vi "Drive Ramp.vi"(8 "Deadband":dbl, 9 "Ramp Value":dbl, 10 "Control Input":dbl, 11 "Previous Value":dbl) -> (3 "Next Value":dbl)   [LabVIEW 2012]
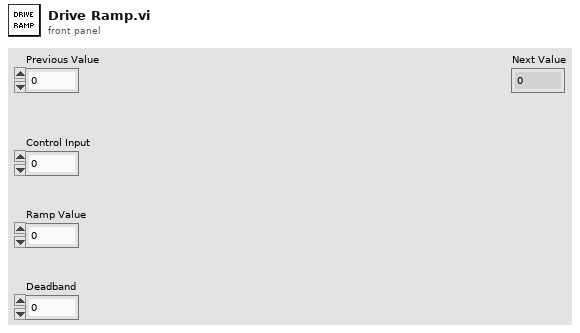
[diagram p1: front panel]
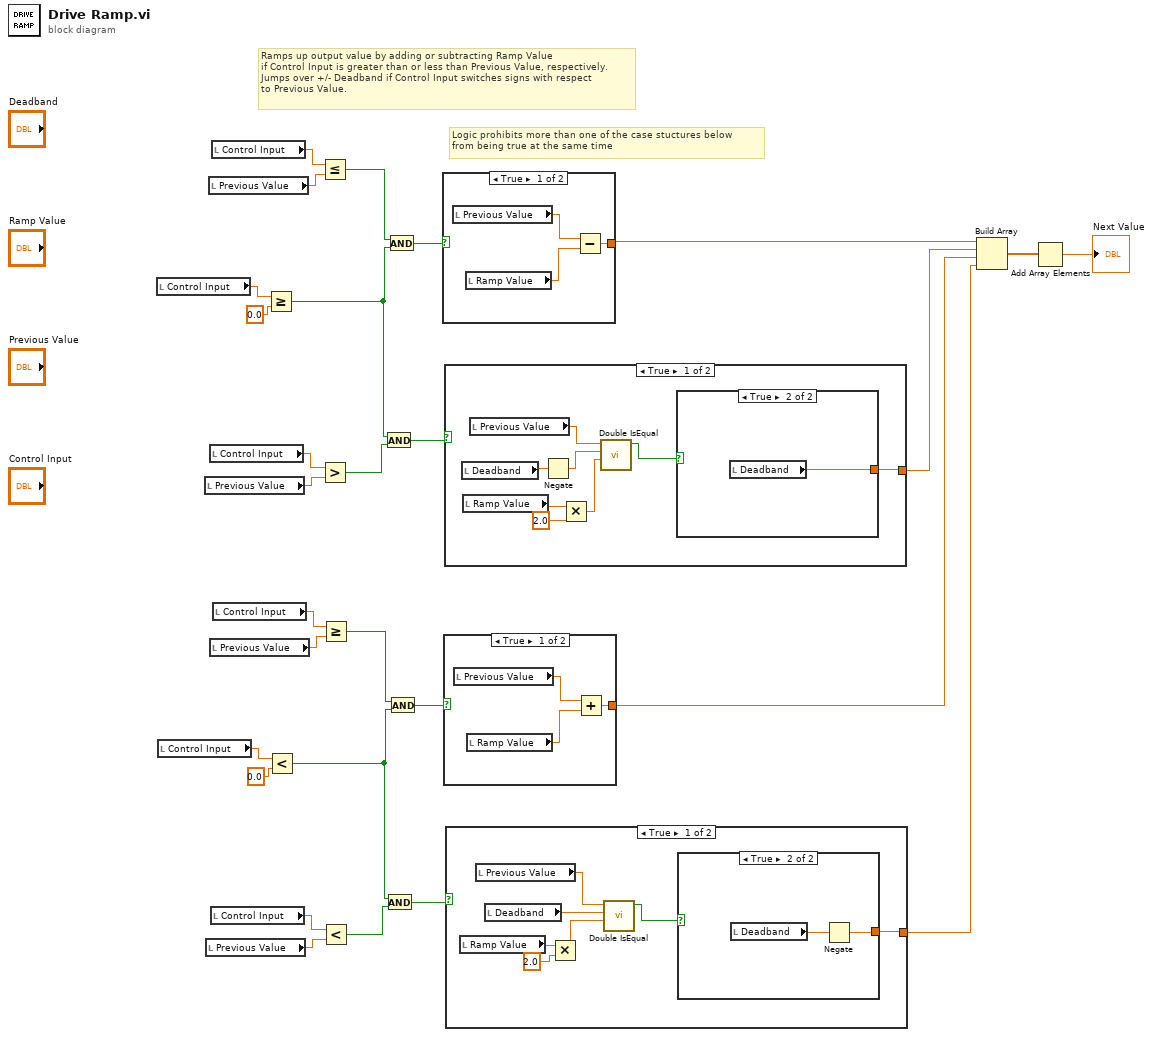
[diagram p0: block diagram]
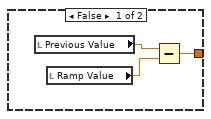
[diagram p2: hidden frame]
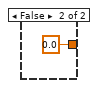
[diagram p3: hidden frame]
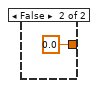
[diagram p4: hidden frame]
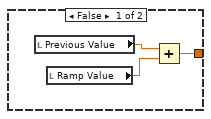
[diagram p5: hidden frame]
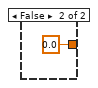
[diagram p6: hidden frame]
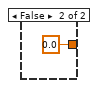
[diagram p7: hidden frame]
diagram:
  # "Logic prohibits more than one of the case stuctures below \nfrom being true at the same time"
  # "Ramps up output value by adding or subtracting Ramp Value\nif Control Input is greater than or less than Previous Value, respectively.\nJumps over +/- Deadband if Control Input switches signs with respect\nto Previous Value."
  n1 = local read "Control Input"() -> (w20:dbl)
  n2 = local read "Control Input"() -> (w9:dbl)
  n3 = local read "Previous Value"() -> (w18:dbl)
  n4 = local read "Previous Value"() -> (w7:dbl)
  n5 = local read "Previous Value"() -> (w22:dbl)
  n6 = local read "Control Input"() -> (w19:dbl)
  n7 = local read "Previous Value"() -> (w11:dbl)
  n8 = local read "Control Input"() -> (w8:dbl)
  n9 = local read "Control Input"() -> (w21:dbl)
  n10 = local read "Control Input"() -> (w10:dbl)
  n11 = Greater Or Equal?(x=w20, y=0.0) -> (x >= y?=w25:bool)
  n12 = Less?(x=w9, y=0.0) -> (x < y?=w14:bool)
  n13 = Less Or Equal?(x=w21, y=w22) -> (x <= y?=w27:bool)
  n14 = Greater?(x=w19, y=w18) -> (0:w24:bool)
  n15 = Greater Or Equal?(x=w10, y=w11) -> (x >= y?=w16:bool)
  n16 = Less?(x=w8, y=w7) -> (x < y?=w13:bool)
  n17 = And(x=w25, y=w24) -> (x .and. y?=w23:bool)
  n18 = And(x=w14, y=w13) -> (x .and. y?=w12:bool)
  n19 = And(x=w27, y=w25) -> (x .and. y?=w26:bool)
  n20 = And(x=w16, y=w14) -> (x .and. y?=w15:bool)
  n21 = case shown="True" w26 {
    tunnel: [w30 0.0] -> w6
    frame True {
      n22 = local read "Previous Value"() -> (w29:dbl)
      n23 = local read "Ramp Value"() -> (w31:dbl)
      n24 = Subtract(x=w29, y=w31) -> (x-y=w30:dbl)
    }
    frame False {
    }
  }
  n25 = case shown="True" w15 {
    tunnel: [w34 0.0] -> w4
    frame True {
      n26 = local read "Previous Value"() -> (w33:dbl)
      n27 = local read "Ramp Value"() -> (w35:dbl)
      n28 = Add(x=w33, y=w35) -> (x+y=w34:dbl)
    }
    frame False {
    }
  }
  n29 = case shown="True" w23 {
    tunnel: [w43 0.0 ("Deadband")] -> w5
    frame True {
      n30 = local read "Deadband"() -> (w44:dbl)
      n31 = local read "Ramp Value"() -> (w42:dbl)
      n32 = local read "Previous Value"() -> (w40:dbl)
      n33 = Negate(x=w44) -> (-x=w39:dbl)
      n34 = Multiply(x=w42, y=2.0) -> (x*y=w38:dbl)
      n35 = call "Double IsEqual.vi"("Epsilon"=w38, "Double2"=w39, "Double1"=w40) -> ("IsEqual"=w37:bool)  [unwired: 8 in]
      n36 = case shown="True" w37 {
        tunnel: [w45 w48] -> w43
        frame False {
          n37 = local read "Previous Value"() -> (w47:dbl)
          n38 = local read "Ramp Value"() -> (w46:dbl)
          n39 = Add(x=w47, y=w46) -> (x+y=w45:dbl)
        }
        frame True {
          n40 = local read "Deadband"() -> (w48:dbl)
        }
      }
    }
    frame False {
    }
  }
  n41 = case shown="True" w12 {
    tunnel: [w56 0.0] -> w3
    frame True {
      n42 = local read "Ramp Value"() -> (w55:dbl)
      n43 = local read "Previous Value"() -> (w53:dbl)
      n44 = local read "Deadband"() -> (w52:dbl)
      n45 = Multiply(x=w55, y=2.0) -> (x*y=w51:dbl)
      n46 = call "Double IsEqual.vi"("Epsilon"=w51, "Double2"=w52, "Double1"=w53) -> ("IsEqual"=w50:bool)  [unwired: 8 in]
      n47 = case shown="True" w50 {
        tunnel: [w57 w61] -> w56
        frame False {
          n48 = local read "Previous Value"() -> (w59:dbl)
          n49 = local read "Ramp Value"() -> (w58:dbl)
          n50 = Subtract(x=w59, y=w58) -> (x-y=w57:dbl)
        }
        frame True {
          n51 = local read "Deadband"() -> (w60:dbl)
          n52 = Negate(x=w60) -> (-x=w61:dbl)
        }
      }
    }
    frame False {
    }
  }
  n53 = Build Array(w6, w5, w4, w3) -> (w2:dbl[])
  n54 = Add Array Elements(numeric array=w2) -> (sum=→"Next Value":dbl)
